vi "Get Transform.vi"(8 "error in (no error)":errorcluster, 9 "Glyph Size":cluster{"Width":sgl, "Height":sgl}, 10 "Canvas Size":cluster{"Width":i32, "Height":i32}, 11 "Transform in":refnum<class "Transform.lvclass">) -> (0 "error out":errorcluster, 1 "Rotation":sgl, 2 "Translation":cluster{"X":sgl, "Y":sgl}, 3 "Transform out":refnum<class "Transform.lvclass">, 4 "Scale":cluster{"X":sgl, "Y":sgl})   [LabVIEW 2020]
uses:
  Transform.lvclass
panel:
  out "new size":cluster{"Width":sgl, "Height":sgl}
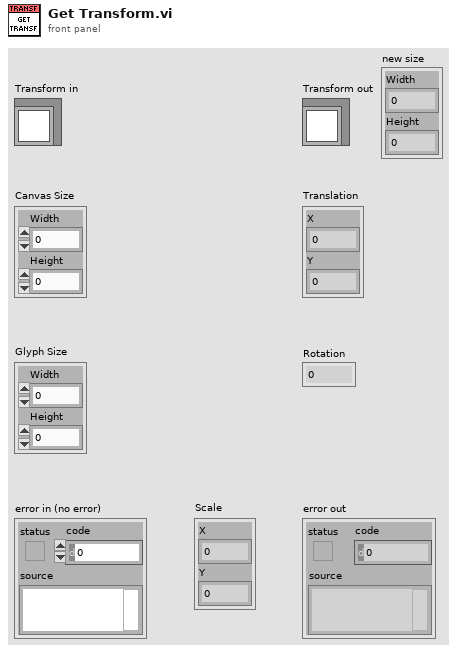
[diagram p1: front panel]
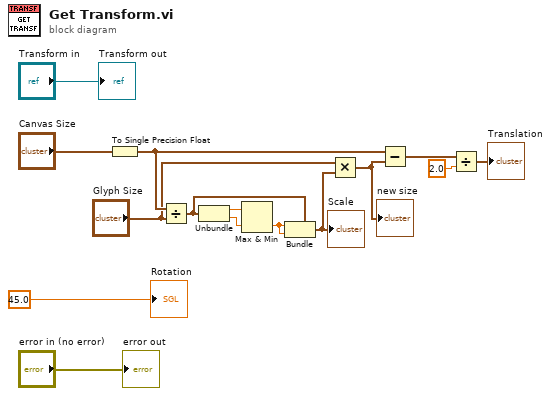
[diagram p0: block diagram]
diagram:
  n1 = To Single Precision Float(number="Canvas Size") -> (single precision float=w9:cluster{"Width":sgl, "Height":sgl})
  n2 = Divide(x=w9, y="Glyph Size") -> (x/y=w7:cluster{"Width":sgl, "Height":sgl})
  n3 = Unbundle(w7) -> ("Width"=w6:sgl, "Height"=w5:sgl)
  n4 = Max & Min(x=w6, y=w5) -> (min(x,y)=w4:sgl)  [unwired: 1 out]
  n5 = Bundle(cluster=w7, "Width"=w4, "Height"=w4) -> (w2:cluster{"Width":sgl, "Height":sgl})
  "Scale" <- w2
  n6 = Multiply(x="Glyph Size", y=w2) -> (x*y=w3:cluster{"Width":sgl, "Height":sgl})
  "new size" <- w3
  n7 = Subtract(x=w9, y=w3) -> (x-y=w11:cluster{"Width":sgl, "Height":sgl})
  n8 = Divide(x=w11, y=sgl 2.0) -> (x/y=→"Translation":cluster{"Width":sgl, "Height":sgl})
  "error out" <- "error in (no error)"
  "Transform out" <- "Transform in"
  "Rotation" <- 45.0 ("Rotation")
